vi "RTT_XCorr_Method (SubVI).vi"(10 "P BWD":waveform(dbl), 11 "P FWD":waveform(dbl)) -> (3 "RTT (ms)":dbl)   [LabVIEW 2017]
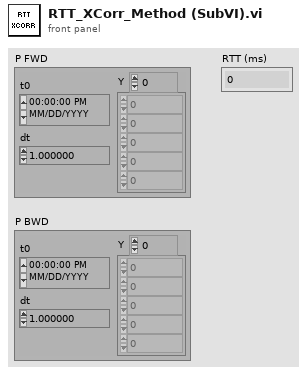
[diagram p1: front panel]
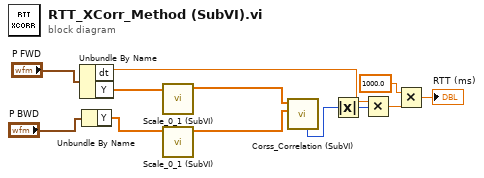
[diagram p0: block diagram]
diagram:
  n1 = Unbundle By Name("P FWD") -> ("dt"=w8:dbl, "Y"=w5:dbl[])
  n2 = Unbundle By Name("P BWD") -> ("Y"=w4:dbl[])
  n3 = call "Scale_0_1 (SubVI).vi"("BLine D"=w5) -> ("Array"=w3:dbl[])  [unwired: 10 in]
  n4 = call "Scale_0_1 (SubVI).vi"("BLine D"=w4) -> ("Array"=w2:dbl[])  [unwired: 10 in]
  n5 = call "Corss_Correlation (SubVI).vi"("Array"=w2, "Array 2"=w3) -> ("M-(N-1)"=w1:i32)  [unwired: 5 in, 4 out]
  n6 = Absolute Value(x=w1) -> (abs(x)=w12:i32)
  n7 = Multiply(x=w8, y=w12) -> (x*y=w9:dbl)
  n8 = Multiply(x=1000.0 ("threshold y"), y=w9) -> (x*y=→"RTT (ms)":dbl)
